vi "Flash Title Bar.vi"(7 "flash time (100)":u32=100, 8 "error in (no error)":errorcluster, 9 "number of flashes (1)":i32=1, 10 "window name (\"\")":string, 11 "window refnum":T1) -> (0 "error out":errorcluster, 3 "window refnum out":T1)   [LabVIEW 2020, in "MacroAssert.lvlib" / "Win Util.lvlib"]
doc: "This function will make the title bar of the window named in the 'window name' input, or identified by the 'window refnum' flash once, the state of the title bar changing at the specified rate the given number of times. If 'not a window refnum' is passed in, then the function will use the window name to get a window window refnum. If the window cannot be found, an error will be returned."
uses:
  Win Util.lvlib
  Window Refnum.ctl
  user32.dll
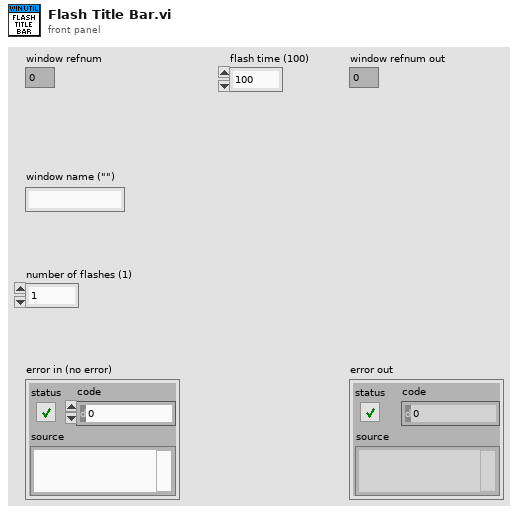
[diagram p1: front panel]
types:
  T1 = typedef "MacroAssert.lvlib/Win Util.lvlib/Window Refnum.ctl" = u64
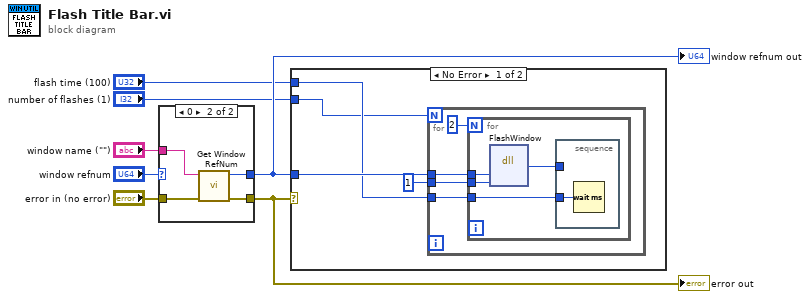
[diagram p0: block diagram]
diagram:
  n1 = case shown="0" "window refnum" {
    selector: "window refnum" -> [w8 _]
    tunnel: "error in (no error)" -> [w9 w13]
    tunnel: [w8 w12] -> w7
    tunnel: [w9 w11] -> w3
    tunnel: "window name (\"\")" -> [_ w10]
    frame Default {
    }
    frame 0 {
      n2 = call "Get Window RefNum.vi"("error in (no error)"=w13, "window name (\"\")"=w10) -> ("error out"=w11:errorcluster, "window refnum (NaWR)"=w12:T1)  [unwired: 6 out]
    }
  }
  "error out" <- w3
  "window refnum out" <- w7
  n3 = case shown="No Error" w3 {
    tunnel: w7 -> [w16 _]
    tunnel: "flash time (100)" -> [w15 _]
    tunnel: "number of flashes (1)" -> [w14 _]
    frame No Error {
      n4 = for {
        N: w14 -> [_]
        tunnel: w15 -> [w20]
        tunnel: 1 -> [w19]
        tunnel: w16 -> [w18]
        n5 = for {
          N: 2 -> [_]
          tunnel: w20 -> [w25]
          tunnel: w19 -> [w24]
          tunnel: w18 -> [w23]
          n6 = dll-call lib="USER32.DLL" fn="FlashWindow"("hWnd"=w23, "fInvert"=w24) -> ("active?"=w22:i32)  [unwired: 5 in, 2 out]
          n7 = stacked-sequence {
            tunnel: w25 -> [w26]
            tunnel: w22 -> [_]
            frame #0 {
              n8 = Wait (ms)(milliseconds to wait=w26) -> ()  [unwired: 1 out]
            }
          }
        }
      }
    }
    frame Error {
    }
  }
